vi "update.vi"(8 "error in (no error)":errorcluster, 11 "ElectrometerController in":refnum<class "ElectrometerController.lvclass">) -> (0 "error out":errorcluster, 1 "newValue":bool, 2 "timeout?":bool, 3 "ElectrometerController out":refnum<class "ElectrometerController.lvclass">, 4 "lastMeasure":T1)   [LabVIEW 2016, in "ElectrometerController.lvclass"]
uses:
  ElectrometerController.lvclass
  ts_electrometeruserevents/Typedefs/Reading.ctl
  <resource>/XMacro.xnode
  Electrometer/State/ElectrometerState.lvclass
  ts_electrometeruserevents/Typedefs/ElectrometerTypedefs.lvlib
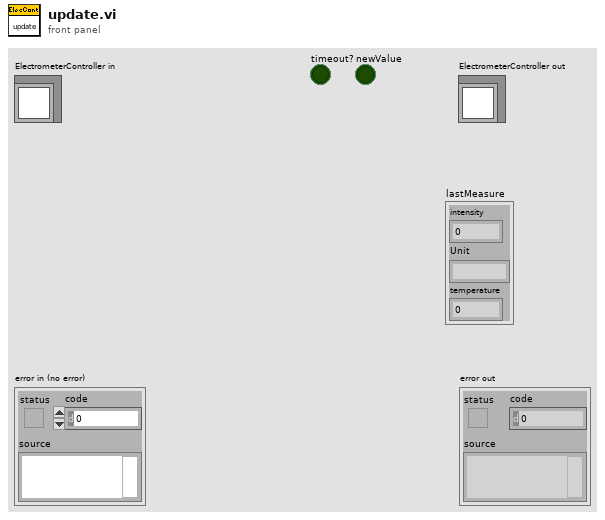
[diagram p1: front panel]
types:
  T1 = typedef "ElectrometerTypedefs.lvlib/Reading.ctl" = cluster{"intensity":dbl, "Unit":string, "temperature":dbl}
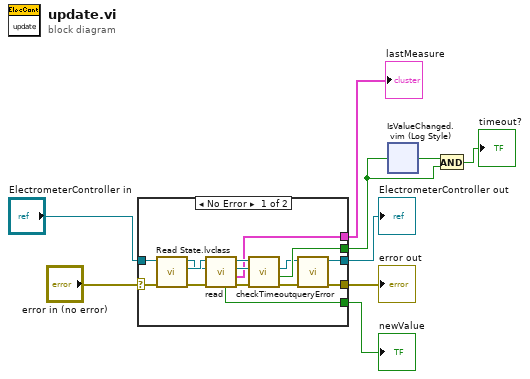
[diagram p0: block diagram]
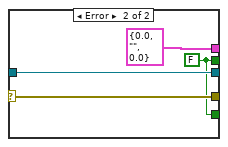
[diagram p2: hidden frame]
diagram:
  n1 = case shown="No Error" "error in (no error)" {
    selector: "error in (no error)" -> [w18 w28]
    tunnel: [w10 w28] -> w8
    tunnel: [w12 w27] -> w6
    tunnel: "ElectrometerController in" -> [w17 w27]
    tunnel: [w16 w26] -> w5
    tunnel: [w15 T1 {"intensity"=0.0, "Unit"="", "temperature"=0.0} ("lastMeasure")] -> w1
    tunnel: [w14 w26] -> w2
    frame No Error {
      n2 = call-dynamic "Read State.lvclass.vi"("error in (no error)"=w18, "ElectrometerController in"=w17) -> ("error out"=w22:errorcluster, "ElectrometerState"=w24:refnum<class "ElectrometerState.lvclass">, "ElectrometerController out"=w23:refnum<class "ElectrometerController.lvclass">)  [unwired: 7 in]
      n3 = call-dynamic "read.vi"("error in (no error)"=w22, "ElectrometerController in"=w23, "State in"=w24) -> ("error out"=w21:errorcluster, "lastMeasure"=w15:T1, "ElectrometerController out"=w20:refnum<class "ElectrometerController.lvclass">, "State out"=w19:refnum<class "ElectrometerState.lvclass">, "newValue"=w16:bool)  [unwired: 4 in]
      n4 = call-dynamic "checkTimeout.vi"("error in (no error)"=w21, "ElectrometerController in"=w20, "State in"=w19) -> ("error out"=w11:errorcluster, "timeout?"=w14:bool, "ElectrometerController out"=w13:refnum<class "ElectrometerController.lvclass">)  [unwired: 5 in, 1 out]
      n5 = call "queryError.vi"("error in (no error)"=w11, "ElectrometerController in"=w13) -> ("error out"=w10:errorcluster, "ElectrometerController out"=w12:refnum<class "ElectrometerController.lvclass">)  [unwired: 7 in, 1 out]
    }
    frame Error {
      w26 = FALSE ("timeout?")
    }
  }
  "error out" <- w8
  "ElectrometerController out" <- w6
  "newValue" <- w5
  "lastMeasure" <- w1
  n6 = xnode "IsValueChanged.vim (Log Style)"("x"=w2) -> ("changed?"=w4:bool)
  n7 = And(x=w4, y=w2) -> (x .and. y?=→"timeout?":bool)
